vi "LS340Monitor.vi"() -> ()   [LabVIEW 2015]
uses:
  Global/Global Variables/Data_Display_global.vi
  Instrument_Setup.vi
  Equipment/Lake Shore Cryotronics 340/Lake Shore Cryotronics 340.lvlib
panel:
  out "SP kleiner als":dbl
  out "Temperature (K)":dbl=291.191
  in  "stop":bool
  in  "VISA session":refnum<visa-resource-name>="GPIB0::12::INSTR"
  out "Temperature":cluster{dbl[], dbl[]}(graph)={[452.667759], [291.191]}
  out "Heater Power":cluster{dbl[], dbl[]}(graph)={[452.667759], [0.0]}
  out "Heater Power (%)":dbl
  out "Heater (%)":dbl(slide) scale=0.0..100.0
  out "Setpoint ITC (K)":dbl=300.0
  out "Offset new SP":dbl
  out "Heater Range":dbl
  out "P (Gain)":dbl
  out "I (Reset)":dbl
  out "D (Rate)":dbl
  in  "Update every [ms]":dbl min=0.0 max=10000.0 step=500.0
  out "HeaterTableLS340.txt":string caption="PID Table"
  in  "Pfad zu HeaterTable":path=path "D:/Cryostat Software/CryoTUM-V1.0/sub_vi-s/Heater Tables/HeaterTableLS340.txt"
  # "0: Off\n1: 10mW\n2: 100mW\n3: 1.0W\n4: 10W"
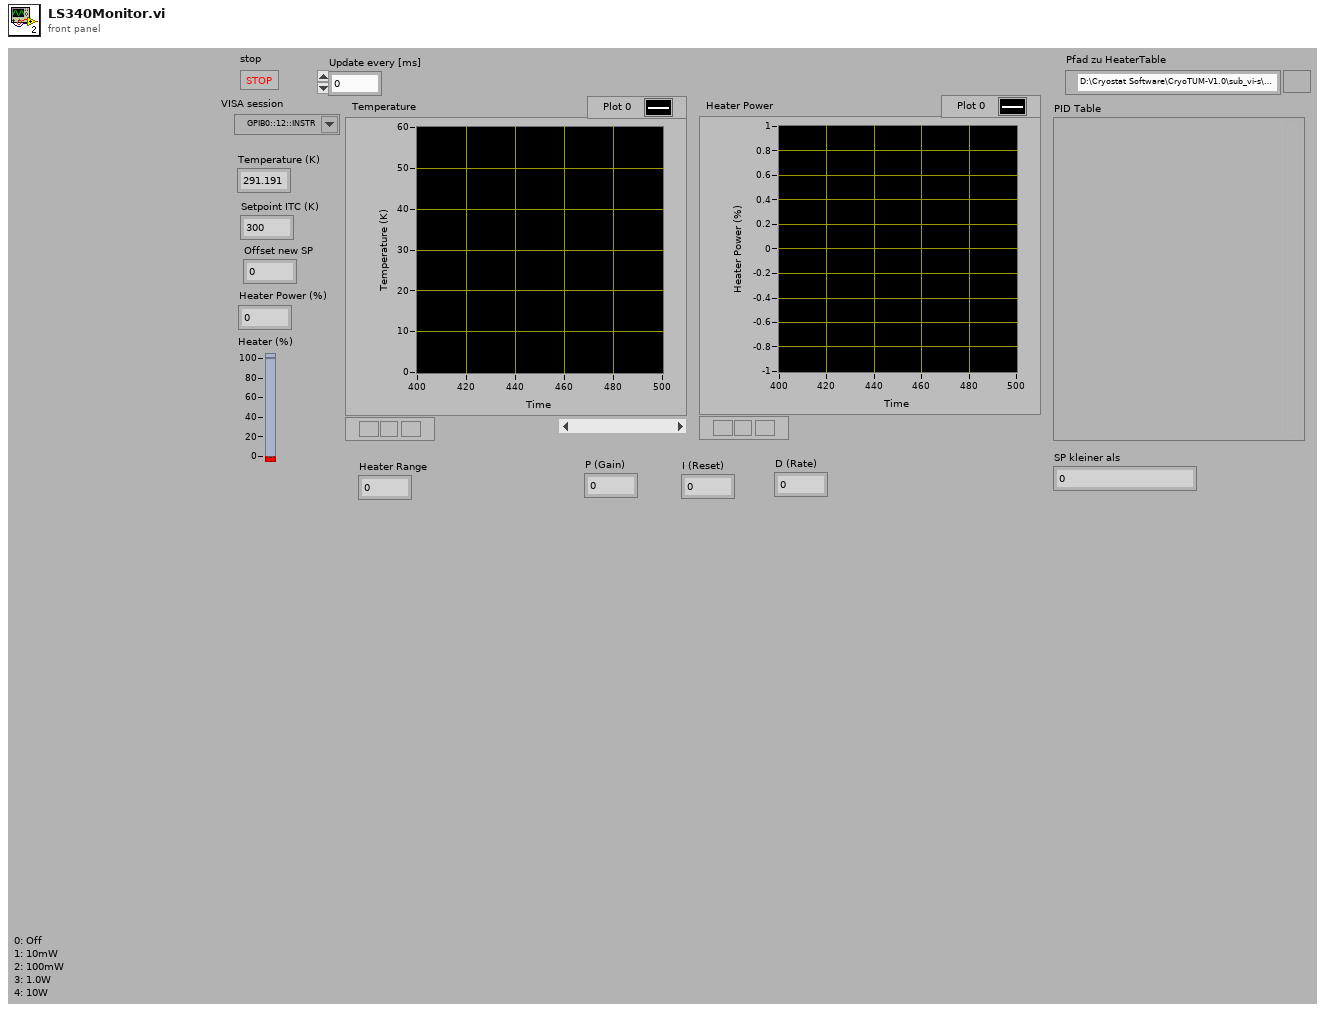
[diagram p1: front panel]
types:
  T1 = enum16{"open", "replace", "create", "open or create", "replace or create", "replace or create with confirmation"}
  T2 = typedef "ITCIO.ctl" = cluster{"Address":T3, "Version":T4, "Ch 1 dec places":i16, "Ch 2 dec places":i16, "Ch 3 dec places":i16, "Ch1 Name":string, "Ch2 Name":string, "Ch3 Name":string}
  T3 = typedef "OxfordAddress.ctl" = cluster{"Com Port":i32, "ISOBUS Address":i32, "GPIB Address":i16, "Communication":enum16{"RS232", "ISOBUS", "GPIB", "Gateway"}}
  T4 = typedef "ITCVersion.ctl" = enum16{"ITC502", "ITC503", "ITC601"}
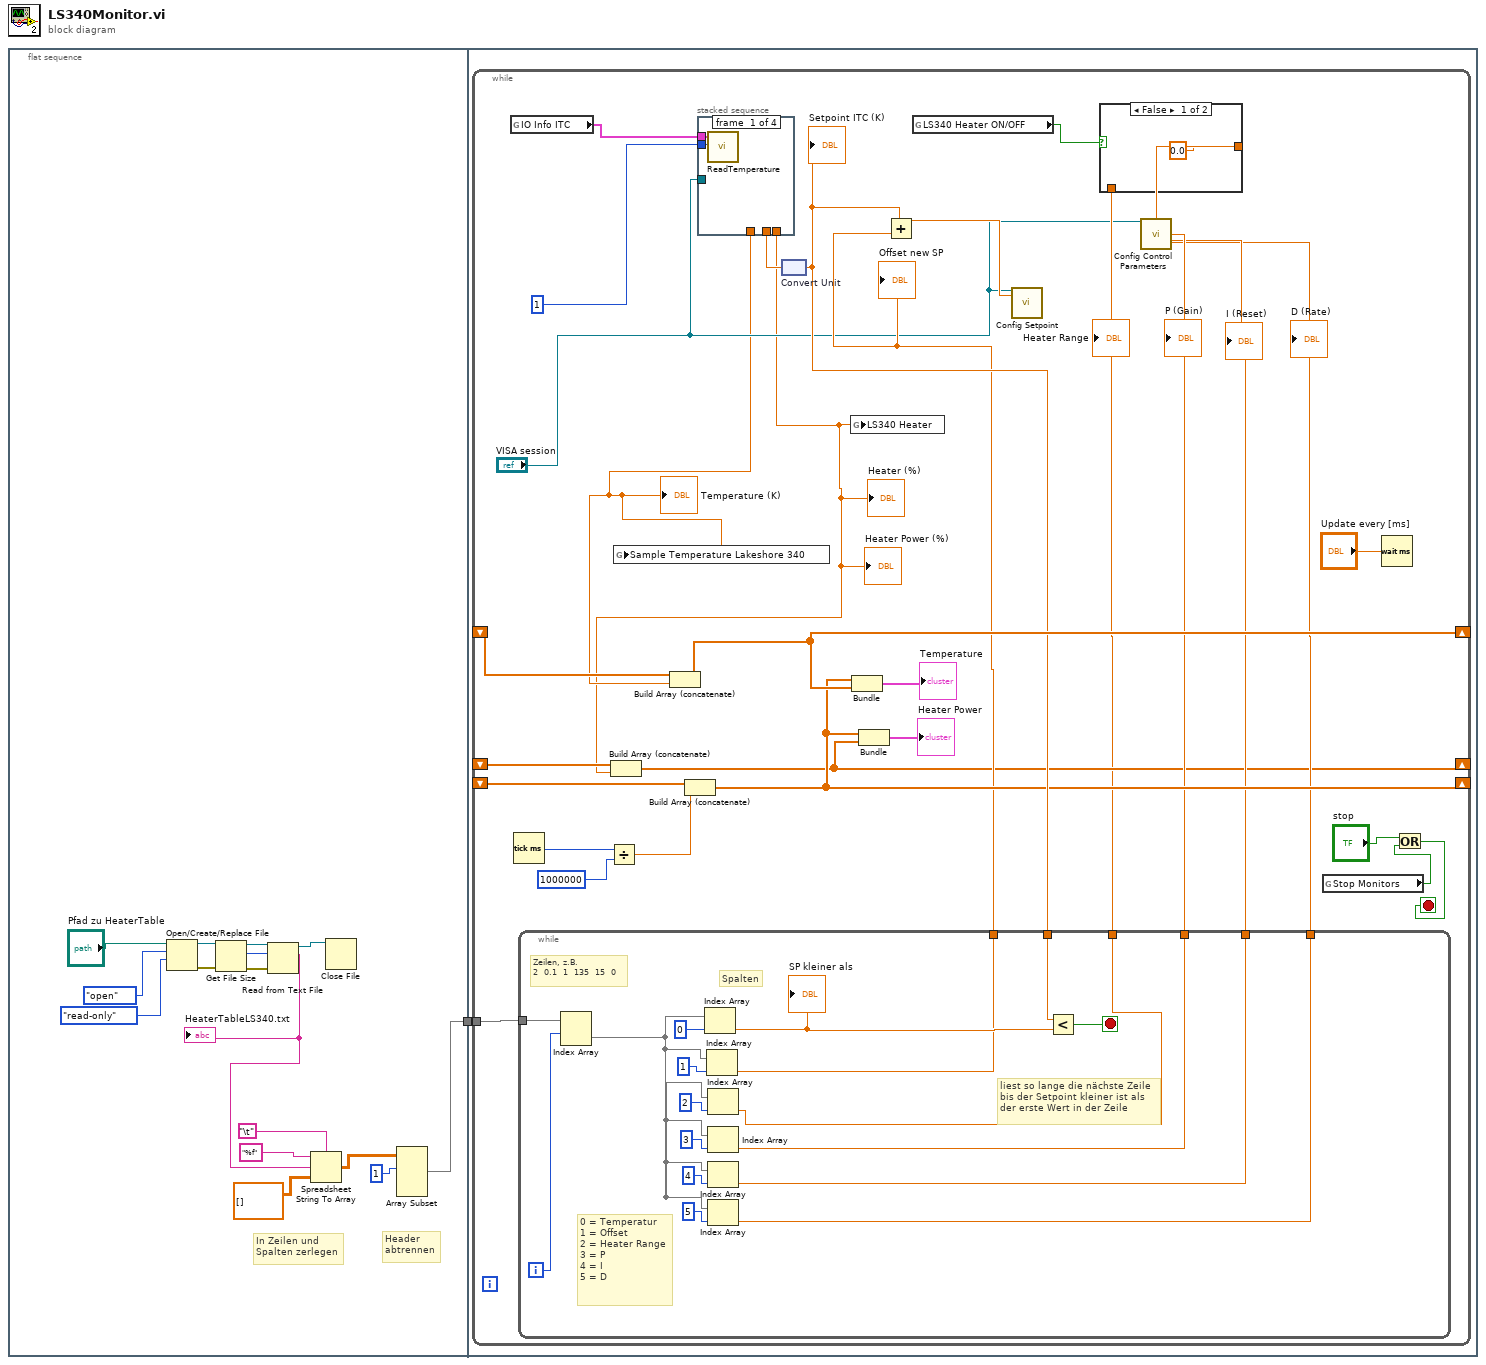
[diagram p0: block diagram]
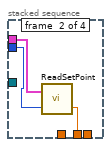
[diagram p2: hidden frame]
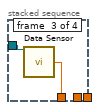
[diagram p3: hidden frame]
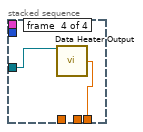
[diagram p4: hidden frame]
diagram:
  n1 = flat-sequence {
    tunnel: [w2] -> w1
    tunnel: w1 -> [w18]
    frame #0 {
      # "In Zeilen und \nSpalten zerlegen"
      # "Header\nabtrennen"
      n2 = Open/Create/Replace File(file path (use dialog)="Pfad zu HeaterTable", operation (0:open)=T1."open", access (0:read/write)=enum16{"read/write", "read-only", "write-only"}."read-only") -> (refnum out=w12:refnum<file>, error out=w14:errorcluster)  [unwired: 3 in, 1 out]
      n3 = Get File Size(file=w12, error in=w14) -> (refnum out=w11:refnum<file>, size (in bytes)=w7:i64, 0:w13:errorcluster)
      n4 = Read from Text File(file (use dialog)=w11, count=w7, error in=w13) -> (refnum out=w10:refnum<file>, text=w6:string)  [unwired: 1 in, 2 out]
      "HeaterTableLS340.txt" <- w6
      n5 = Spreadsheet String To Array(delimiter (Tab)="\t", format string="%f", spreadsheet string=w6, array type (2D Dbl)=dbl[][] []) -> (array=w5:dbl[][])
      n6 = Close File(refnum=w10) -> ()  [unwired: 1 in, 2 out]
      n7 = Array Subset(array=w5, index (row)=1) -> (w2:dbl[][])  [unwired: 3 in]
    }
    frame #1 {
      n8 = while {
        shift-right: [w41] -> _
        shift-left: _ -> [w42]
        shift-right: [w31] -> _
        shift-left: _ -> [w49]
        shift-right: [w36] -> _
        shift-left: _ -> [w48]
        tunnel: w18 -> [w39]
        stop <- w26 stop-if-true
        n9 = global read "Instrument_Setup.vi" "IO Info ITC"() -> (w24:T2)
        n10 = Tick Count (ms)() -> (millisecond timer value=w45:u32)
        n11 = Divide(x=w45, y=u32 1000000 ("milliseconds to wait")) -> (x/y=w44:dbl)
        n12 = Build Array (concatenate)(w48, w44) -> (w36:dbl[])
        n13 = stacked-sequence {
          tunnel: w24 -> [w51 w53 _ _]
          tunnel: 1 -> [w50 w52 _ _]
          tunnel: [_ w54 _ _] -> w23
          tunnel: "VISA session" -> [_ _ w56 w58]
          tunnel: [_ _ w55 _] -> w20
          tunnel: [_ _ _ w57] -> w19
          frame #0 {
            n14 = call "ReadTemperature.vi"("Channel"=w50, "IO Info"=w51) -> ()  [unwired: 3 in, 3 out]
          }
          frame #1 {
            n15 = call "ReadSetPoint.vi"("Control Ch"=w52, "IO Info"=w53) -> ("Set point"=w54:dbl[unit])  [unwired: 1 out]
          }
          frame #2 {
            n16 = call "Data Sensor.vi"("VISA resource name"=w56) -> ("Kelvin Reading"=w55:dbl)  [unwired: 10 in, 4 out]
          }
          frame #3 {
            n17 = call "Data Heater Output.vi"("VISA resource name"=w58) -> ("Heater Output"=w57:dbl)  [unwired: 12 in, 2 out]
          }
        }
        "Temperature (K)" <- w20
        "Heater Power (%)" <- w19
        "Heater (%)" <- w19
        n18 = Build Array (concatenate)(w49, w19) -> (w31:dbl[])
        n19 = global write "Data_Display_global.vi" "Sample Temperature Lakeshore 340"(w20) -> ()
        n20 = Build Array (concatenate)(w42, w20) -> (w41:dbl[])
        n21 = node "Convert Unit"(w23) -> (w38:dbl)
        "Setpoint ITC (K)" <- w38
        n22 = while {
          tunnel: w39 -> [w77]
          tunnel: w38 -> [w67]
          tunnel: [w66] -> w35
          tunnel: [w64] -> w30
          tunnel: [w63] -> w34
          tunnel: [w62] -> w33
          tunnel: [w61] -> w32
          i -> [w76]
          stop <- w69 stop-if-true
          # "0 = Temperatur\n1 = Offset\n2 = Heater Range\n3 = P\n4 = I\n5 = D"
          # "liest so lange die nächste Zeile\nbis der Setpoint kleiner ist als \nder erste Wert in der Zeile"
          # "Zeilen, z.B. \n2  0.1  1  135  15  0"
          # "Spalten"
          n23 = Index Array(array=w77, index (row)=w76) -> (element=w70:dbl[])  [unwired: 1 in]
          n24 = Index Array(array=w70, index=0) -> (element=w68:dbl)
          "SP kleiner als" <- w68
          n25 = Index Array(array=w70, index=1) -> (element=w66:dbl)
          n26 = Index Array(array=w70, index=2) -> (element=w64:dbl)
          n27 = Index Array(array=w70, index=3) -> (element=w63:dbl)
          n28 = Index Array(array=w70, index=4) -> (element=w62:dbl)
          n29 = Index Array(array=w70, index=5) -> (element=w61:dbl)
          n30 = Less?(x=w67, y=w68) -> (x < y?=w69:bool)
        }
        "Offset new SP" <- w35
        "Heater Range" <- w30
        "P (Gain)" <- w34
        "I (Reset)" <- w33
        "D (Rate)" <- w32
        n31 = global write "Data_Display_global.vi" "LS340 Heater"(w19) -> ()
        n32 = Bundle(w36, w41) -> (→"Temperature":cluster{dbl[], dbl[]})  [unwired: 1 in]
        n33 = Bundle(w36, w31) -> (→"Heater Power":cluster{dbl[], dbl[]})  [unwired: 1 in]
        n34 = Add(x=w38, y=w35) -> (x+y=w37:dbl)
        n35 = global read "Data_Display_global.vi" "LS340 Heater ON/OFF"() -> (w25:bool)
        n36 = call "Config Setpoint.vi"("VISA resource name"="VISA session", "Setpoint (0.0)"=w37) -> ()  [unwired: 12 in, 2 out]
        n37 = case shown="False" w25 {
          tunnel: w30 -> [_ w60]
          tunnel: [0.0 w60] -> w29
          frame False {
          }
          frame True {
          }
        }
        n38 = call "Config Control Parameters.vi"("VISA resource name"="VISA session", "Heater Range (0: Off)"=w29, "Gain (P) (0.0)"=w34, "Reset (I) (0.0)"=w33, "Rate (D) (0)"=w32) -> ()  [unwired: 9 in, 2 out]
        n39 = global read "Data_Display_global.vi" "Stop Monitors"() -> (w28:bool)
        n40 = Wait (ms)(milliseconds to wait="Update every [ms]") -> ()  [unwired: 1 out]
        n41 = Or(x="stop", y=w28) -> (x .or. y?=w26:bool)
      }
    }
  }
